vi "get_internet_version.vi"(8 "error in (no error)":errorcluster, 11 "HelioUpdateMH100803 in":refnum<class "HelioUpdateMH100803.lvclass">) -> (0 "error out":errorcluster, 3 "HelioUpdateMH100803 out":refnum<class "HelioUpdateMH100803.lvclass">, 4 "version number failed":bool, 5 "internet version out":string)   [LabVIEW 2010, in "HelioUpdateMH100803.lvclass"]
uses:
  HelioUpdateMH100803.lvclass
  HelioUpdateMH100803.lvclass/HelioUpdateMH100803.ctl
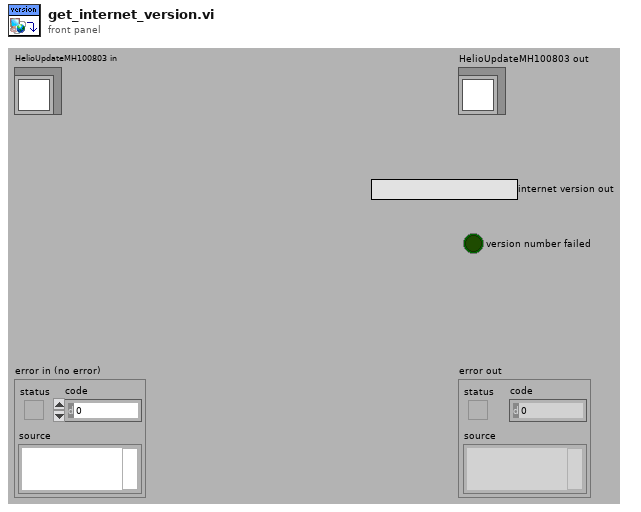
[diagram p1: front panel]
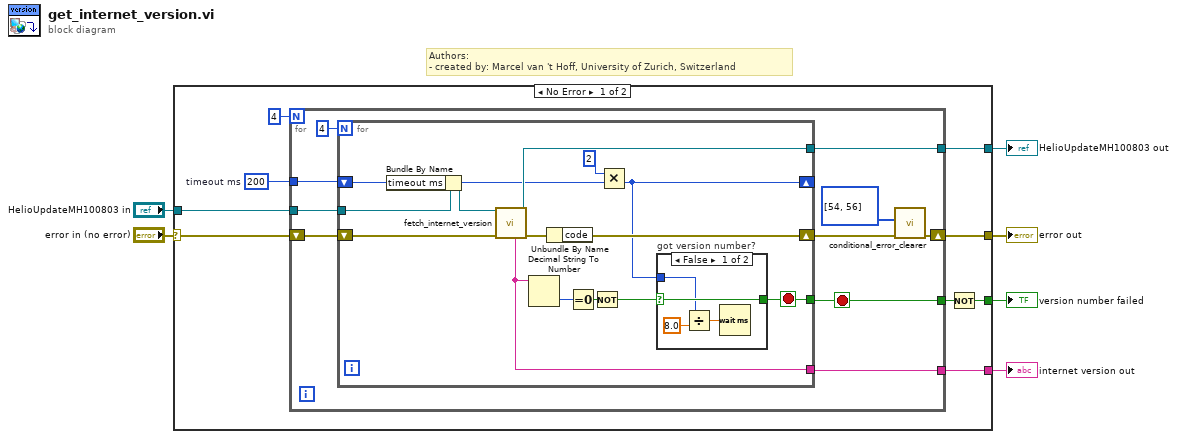
[diagram p0: block diagram]
diagram:
  # "Authors: \n- created by: Marcel van 't Hoff, University of Zurich, Switzerland"
  n1 = case shown="No Error" "error in (no error)" {
    selector: "error in (no error)" -> [w15 w44]
    tunnel: [w7 w44] -> w4
    tunnel: "HelioUpdateMH100803 in" -> [w12 w45]
    tunnel: [w14 w45] -> w3
    tunnel: [w13 _] -> w2
    tunnel: [w8 _] -> w1
    frame No Error {
      w9 = 200  # timeout ms
      n2 = for {
        N: 4 -> [_]
        tunnel: [w19] -> w14
        tunnel: [w24] -> w13
        tunnel: w12 -> [w23]
        tunnel: [w21] -> w10
        tunnel: w9 -> [w20]
        shift-right: [w16] -> w7
        shift-left: w15 -> [w25]
        stop <- w21 stop-if-true
        n3 = for {
          N: 4 -> [_]
          tunnel: [w37] -> w19
          tunnel: [w30] -> w24
          tunnel: w23 -> [w36]
          shift-right: [w28] -> _
          shift-left: w20 -> [w32]
          tunnel: [w31] -> w21
          shift-right: [w34] -> w17
          shift-left: w25 -> [w38]
          stop <- w31 stop-if-true
          n4 = Bundle By Name(cluster=w36, "timeout ms"=w32) -> (w35:refnum<class "HelioUpdateMH100803.lvclass">)
          n5 = call-dynamic "fetch_internet_version.vi"("error in (no error)"=w38, "HelioUpdateMH100803 in"=w35) -> ("error out"=w34:errorcluster, "HelioUpdateMH100803 out"=w37:refnum<class "HelioUpdateMH100803.lvclass">, "internet version out"=w30:string)  [unwired: 7 in]
          n6 = Decimal String To Number(string=w30) -> (number=w29:i32)  [unwired: 2 in, 1 out]
          n7 = Unbundle By Name(w34) -> ()  [unwired: 1 out]
          n8 = Equal To 0?(x=w29) -> (x = 0?=w27:bool)
          n9 = Not(x=w27) -> (.not. x?=w26:bool)
          n10 = Multiply(x=2, y=w32) -> (x*y=w28:i32)
          n11 = case "got version number?" shown="False" w26 {
            selector: w26 -> [w42 w43]
            tunnel: [w42 w43] -> w31
            tunnel: w28 -> [w41 _]
            frame False {
              n12 = Divide(x=w41, y=8.0) -> (x/y=w39:dbl)
              n13 = Wait (ms)(milliseconds to wait=w39) -> ()  [unwired: 1 out]
            }
            frame True {
            }
          }
        }
        n14 = call "conditional_error_clearer.vi"("error in (no error)"=w17, "array of clearable error codes"=i32[] [54, 56]) -> ("error out"=w16:errorcluster)  [unwired: 9 in]
      }
      n15 = Not(x=w10) -> (.not. x?=w8:bool)
    }
    frame Error {
    }
  }
  "error out" <- w4
  "HelioUpdateMH100803 out" <- w3
  "internet version out" <- w2
  "version number failed" <- w1
